vi "Saccade suppression - continuous flash LED by time.vi"() -> ()   [LabVIEW 2013]
uses:
  <vilib>/Platform/TimedLoop/XDataNode/timing_clust.ctl
  <vilib>/Platform/TimedLoop/XDataNode/nitl_modes.ctl
  <vilib>/Platform/TimedLoop/XDataNode/wakeup.ctl
  <vilib>/gmath/statdist.llb/Uniform (Discrete) Random.vi
  Eye tracking dependencies/Global 1.vi
  <vilib>/platform/TimedLoop/XDataNode/XDataNode.xnode
  <vilib>/Platform/TimedLoop/XDataNode/XDNodeRunTimeDep.lvlib
  <vilib>/gmath/NI_Gmath.lvlib
panel:
  out "Eye tracker":bool
  out "Std name":string="70915_animal15-21_exp1"
  out "Blank":bool
  out "Total number of trials":i32=1
  out "Running!":bool
  in  "Location":string="F:\\Beh_Data\\"
  out "File name exists!":bool
  out "Current trial #":u16=1
  out "LED":bool
  in  "Abort":bool caption="run-stop"
  in  "File name":string="18-137_flash"
  in  "Save data":bool
  out "State Missed":bool
  out "VS missed":bool
  out "State busy":bool
  out "VS busy":bool
  in  "Tab Control":T1(tab)=enum."VS Parameters"
  in  "Notes":string
  in  "Start recording @":string
  in  "Inserted probe @":string
  in  "Brain region":string
  in  "Anesthesia @":string
  in  "Anesthesia":string
  in  "Probe configuration":string
  in  "Probe use number":string
  in  "Probe ID":string
  in  "Probe type":string
  in  "Electrode spacing":string
  in  "Electrode area":string
  in  "Penetration angle (to pia)":string
  in  "Penetration coordinates":string
  in  "Penetration distance":string
  in  "Penetration number":string
  in  "Genotype":string
  in  "Transfection":string
  in  "Mass":string
  in  "Sex":string
  in  "Age":string
  in  "Animal ID":string="14-4"
  in  "inter flash interval (ms)":dbl=6000.0
  in  "Max jitter (ms)":dbl=500.0
  in  "VS type":string="saccade_grating"
  in  "Background luminance":sgl=60.0
  in  "Pulse amp 0":sgl
  in  "Pulse amp 1":sgl
  in  "Pulse delay (ms)":sgl
  in  "Pulse width (ms)":sgl
  in  "Pulse period":sgl
  in  "Pulse #":sgl
  in  "LED mode":u16(ring) items=["No LED", "Random"]
  in  "Chance (%)":dbl
  in  "# of trials":i32=1
  in  "run-stop":bool
  in  "Time (min)":sgl=5.0
  in  "Flash luminance":sgl=100.0
  in  "flash duration (ms)":dbl=16.0
  in  "VS subtype":string="shiftByTime2"
  in  "Include blanks":bool
  in  "# of blank trials":i32=6
  in  "INTERLEAVE BLANKS":bool
  in  "Give reward":bool
  in  "Manually give shock":bool
  in  "Water duration (ms)":u32=30
  in  "Shock duration (ms)":u32=10
  in  "Water refractory period (ms)":u32=500
  in  "Shock refractory period (ms)":u32=1000
  in  "Trial timeout (ms)":u32=3000
  in  "Track eye":bool=TRUE
  in  "Allow shock":bool
  in  "Allow timeout":bool
  in  "Manually give water":bool
  in  "Reward period (ms)":u32
  in  "Reward start delay (ms)":u32
  in  "Lick threshold (V)":fxp<+,32,16>=1.600006103515625
  in  "VS threshold (V)":fxp<+,32,16>=2.0
  out "Originating IP":string="192.168.137.2"
  out "Incoming data":string="TrlDone 1.000 "
  in  "Update cycle (ms)":dbl=50.0
  in  "Local IP_This computer":string="192.168.137.10"
  in  "Remote IP_Broadcast":string="192.168.137.255"
  in  "Remote IP_State machine":string="192.168.137.2"
  in  "Remote IP_Visual stimulation":string="192.168.137.3"
  in  "Local port":u16=9090
  in  "Remote port":u16=9091
  out "Error 2":string
  # "Saccade suppression project"
  # "Current trial"
  # "of"
  # "System Status"
  # "VS"
  # "State machine"
  # "Busy"
  # "Missed trial"
  # "Max 20 characters"
  # "(w/o LED)"
  # "Alt: saccade_grating"
  # "Alt: continuous_flash"
  # "movingByTime"
  # "stripeFlipByTime"
  # "gratingFlipByTime"
  # "Time per trial (min)"
  # "MAX 199.9988"
  # "(% of blank trials that have LED)"
  # "Alt: saccade_grating"
  # "shiftByTime"
  # "Errors for debugging"
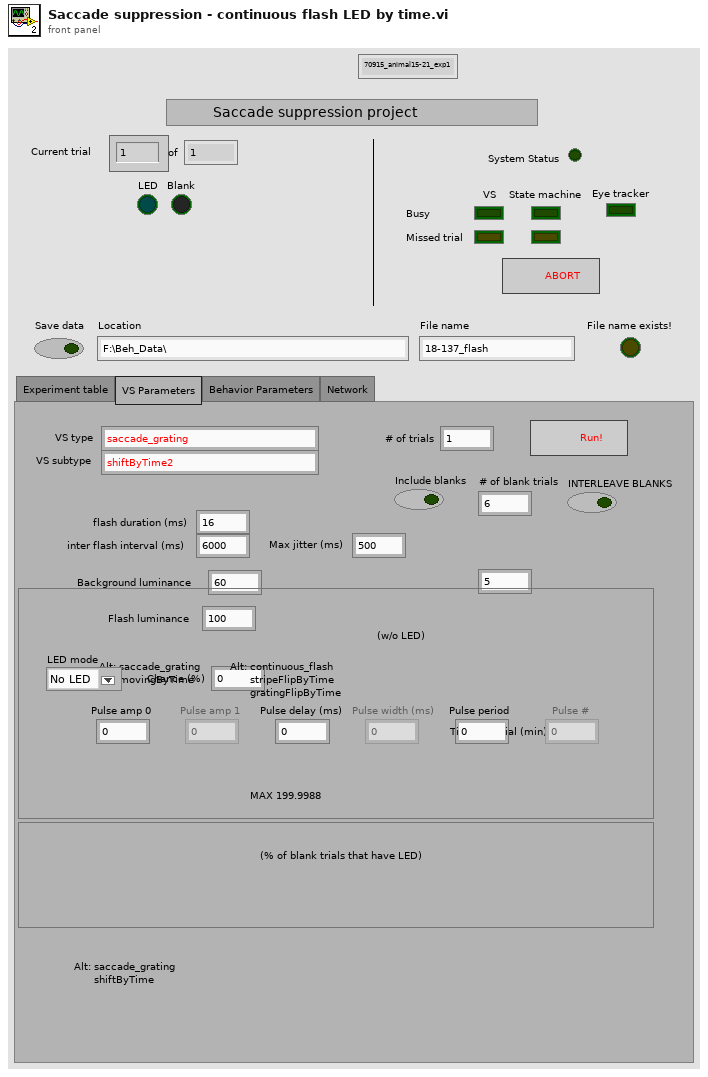
[diagram p1: front panel]
types:
  T1 = enum32{"Experiment table", "VS Parameters", "Behavior Parameters", "Network"}
  T2 = typedef "XDNodeRunTimeDep.lvlib/timing_clust.ctl" = cluster{"Expected End [f-1]":u64, "Actual End [f-1]":u64, "Finished Late? [f-1]":bool, "Expected End [i-1]":u64, "Actual End [i-1]":u64, "Finished Late? [i-1]":bool, "Expected Start [i]":u64, "Actual Start [i]":u64, "Expected Start [f]":u64, "Actual Start [f]":u64, "Source Name":string, "Structure Name":string, "Period":i64, "Deadline":i64, "Offset":i64, "Start":i64, "Priority":i32, "Timeout":i32, "Mode":T3, "Wakeup Reason":T4, "Error":errorcluster, "Source Type":string, "Secondary Source Type":string, "Global End Time":u64, "Global Start Time":u64, "Frame Duration":u64, "Iteration Duration":u64, "Assigned CPU":i32, "I/O Scan Engine Mode":u32}
  T3 = typedef "XDNodeRunTimeDep.lvlib/nitl_modes.ctl" = enum32{"No Change", "Process missed periods, maintain original phase", "Discard missed periods, maintain original phase", "Process missed periods, ignore original phase", "Discard missed periods, ignore original phase"}
  T4 = typedef "XDNodeRunTimeDep.lvlib/wakeup.ctl" = enum32{"Normal", "Aborted", "Asynchronous wakeup", "Timing source error", "Timed loop error", "Timeout"}
  T5 = enum16{"big-endian, network order", "native, host order", "little-endian"}
  T6 = enum16{"open", "replace", "create", "open or create", "replace or create", "replace or create with confirmation"}
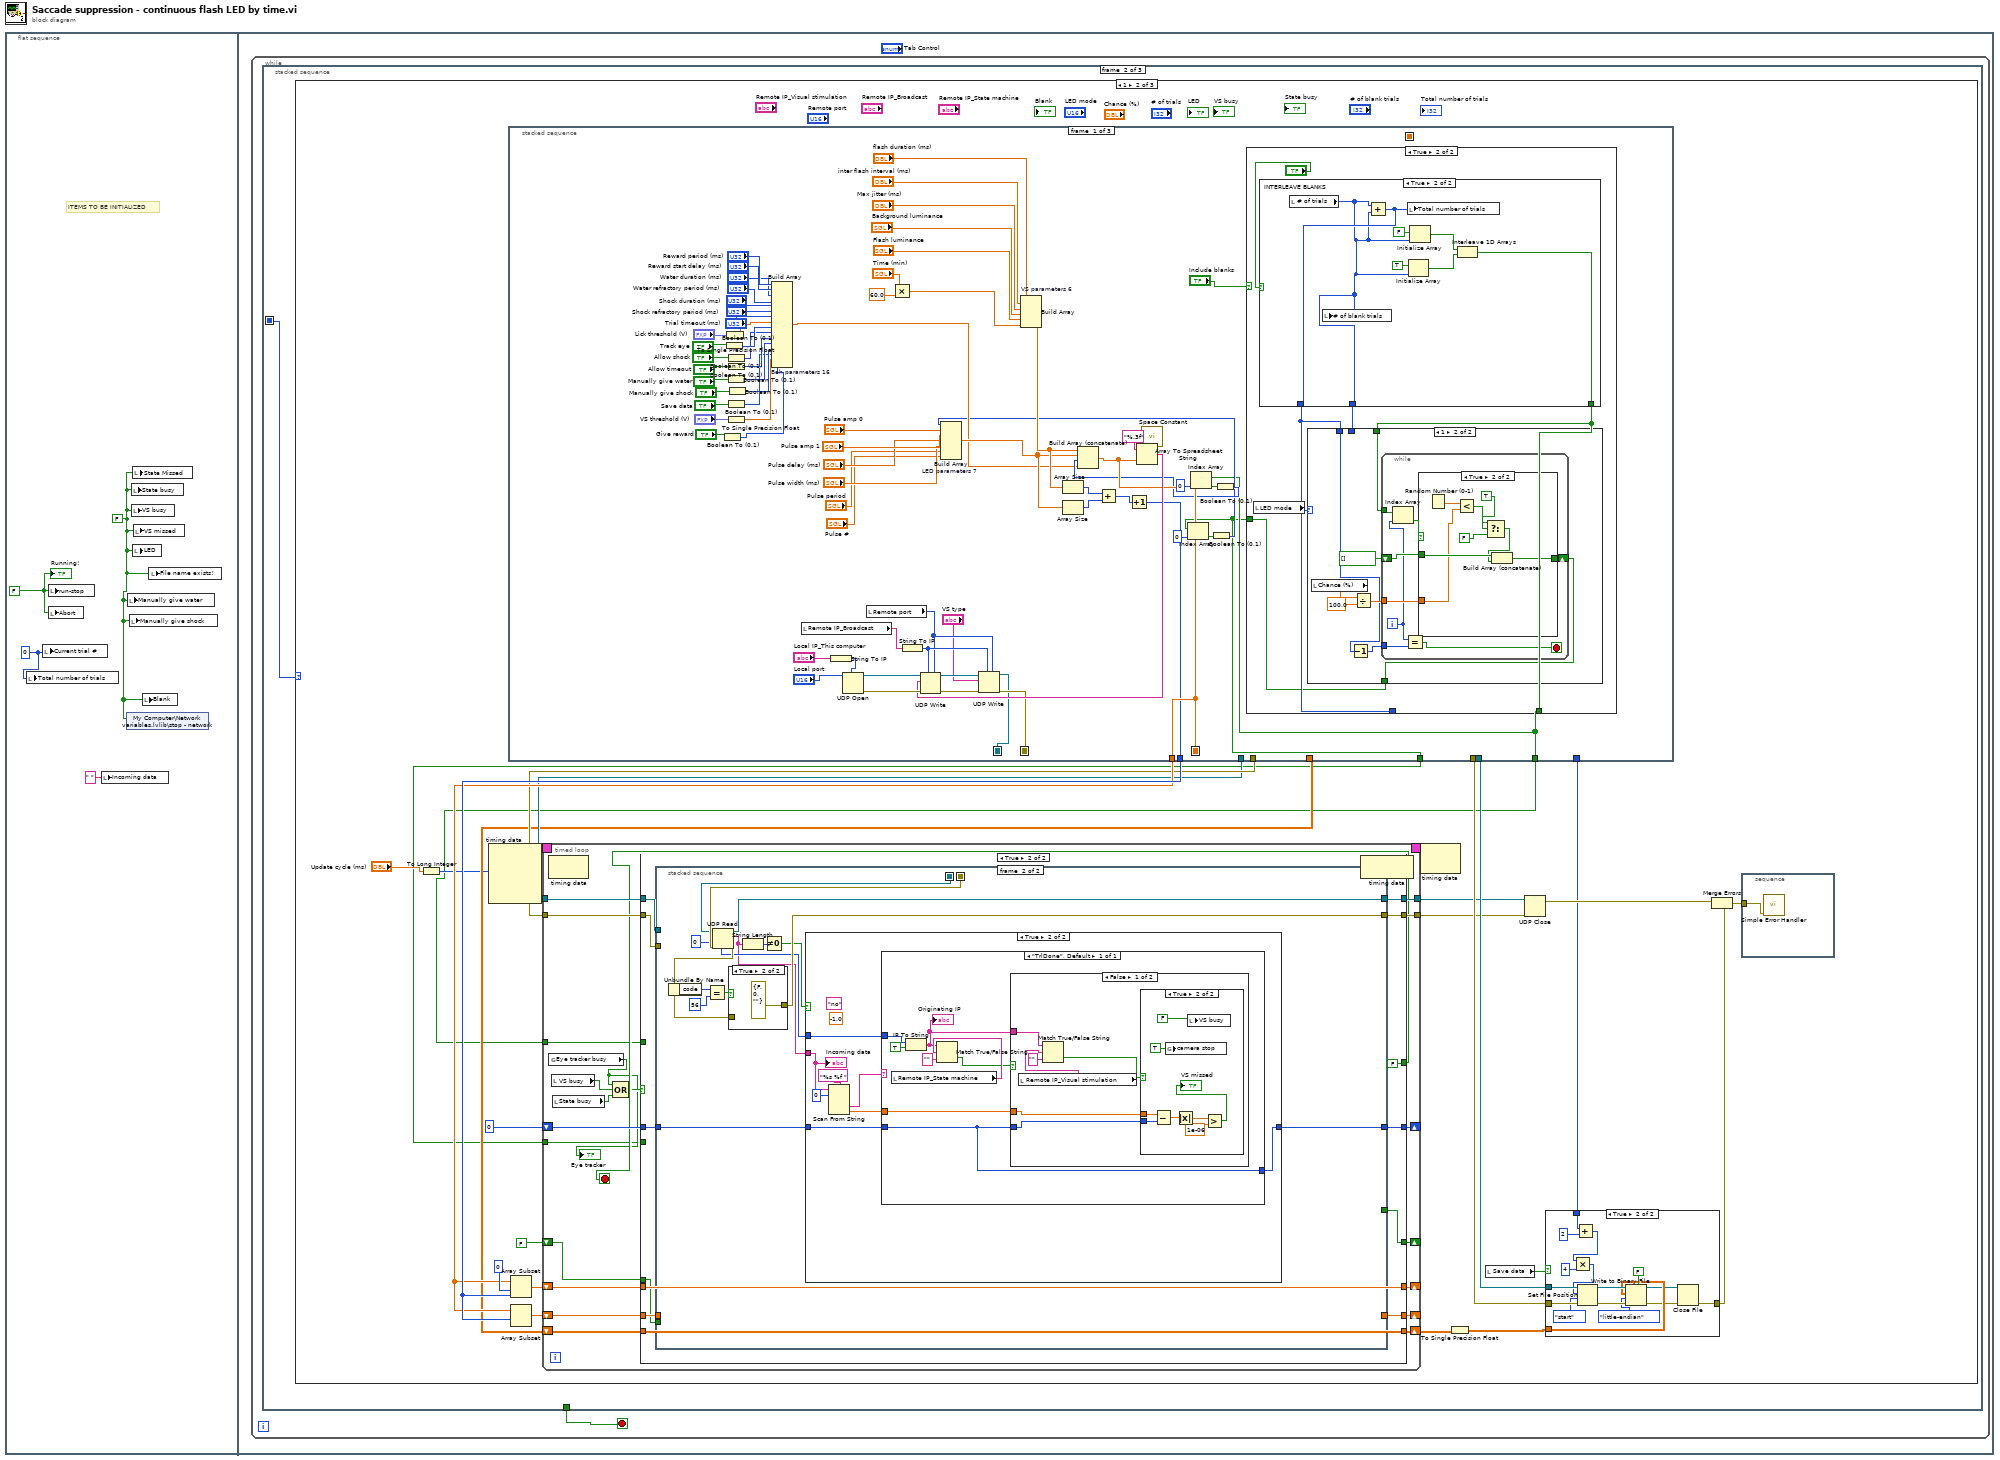
[diagram p0: block diagram]
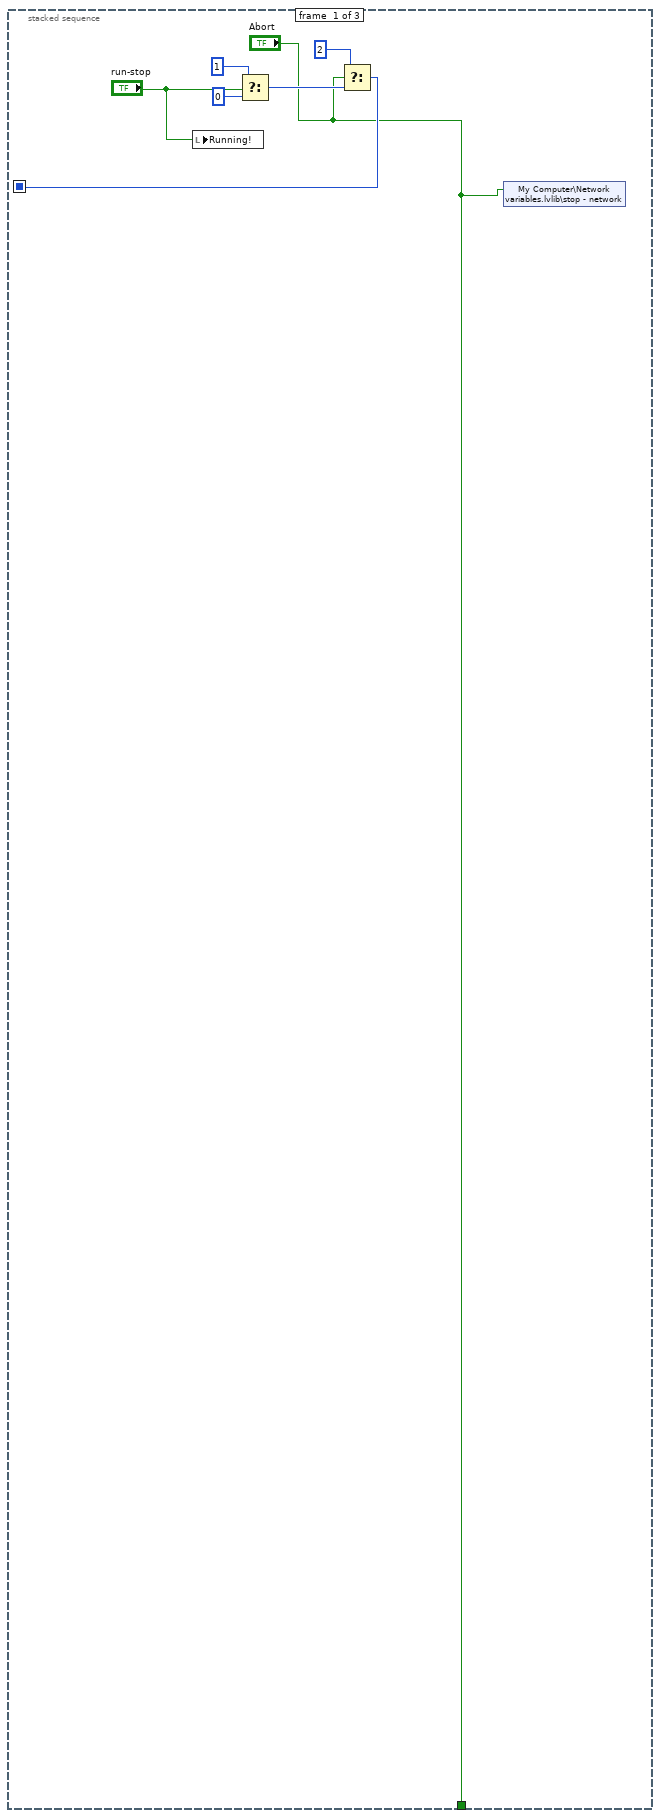
[diagram p2: hidden frame]
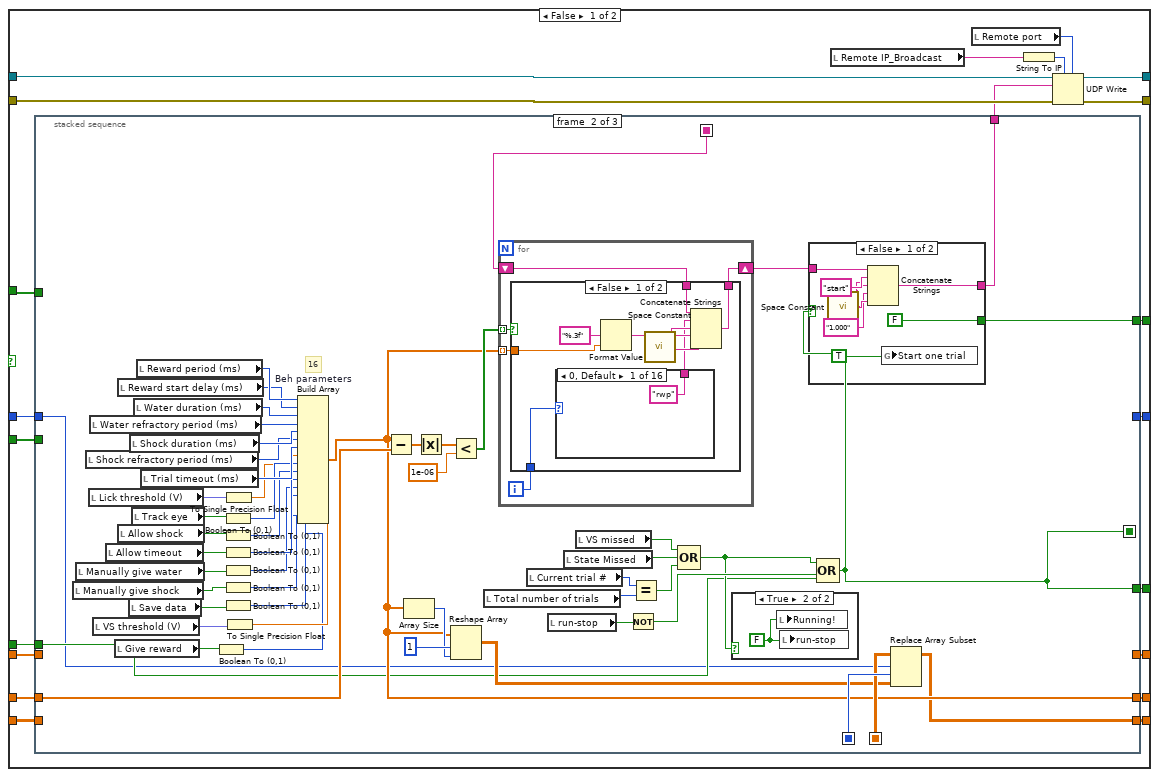
[diagram p4: hidden frame]
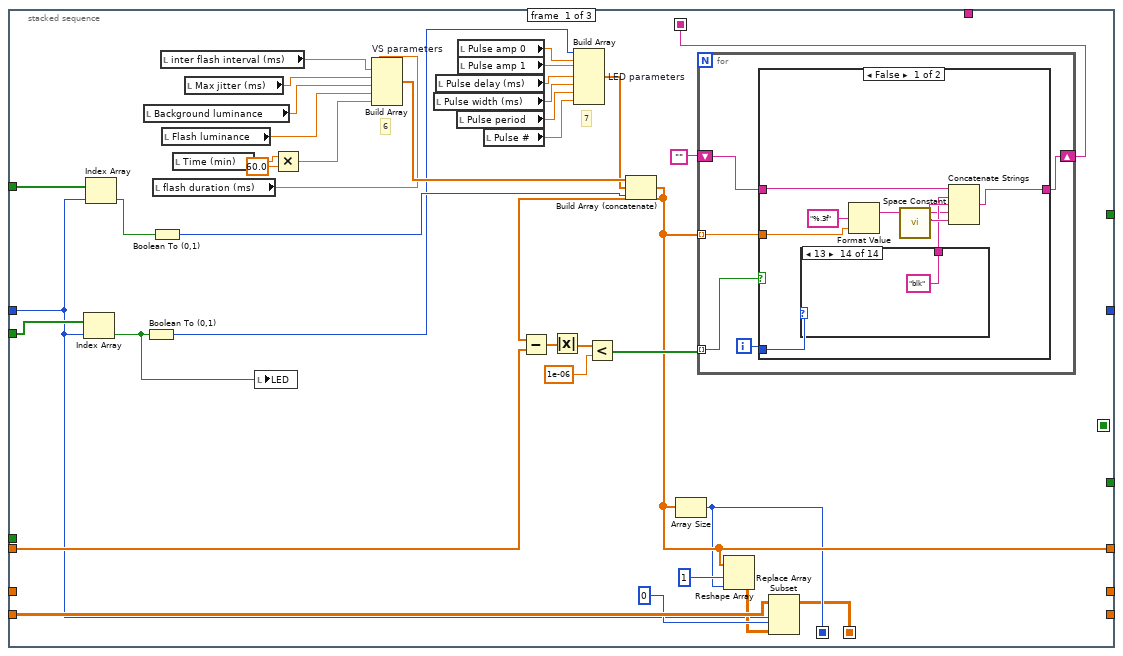
[diagram p5: hidden frame]
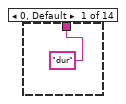
[diagram p6: hidden frame]
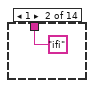
[diagram p7: hidden frame]
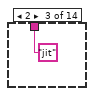
[diagram p8: hidden frame]
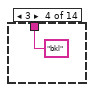
[diagram p9: hidden frame]
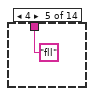
[diagram p10: hidden frame]
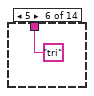
[diagram p11: hidden frame]
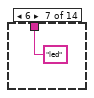
[diagram p12: hidden frame]
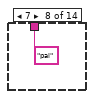
[diagram p13: hidden frame]
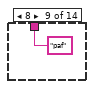
[diagram p14: hidden frame]
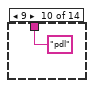
[diagram p15: hidden frame]
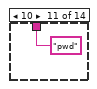
[diagram p16: hidden frame]
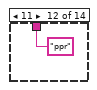
[diagram p17: hidden frame]
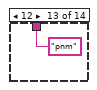
[diagram p18: hidden frame]
diagram:
  n1 = flat-sequence {
    frame #0 {
      w3 = u16 0
      w2 = FALSE ("L dist ind")
      w4 = FALSE
      # "ITEMS TO BE INITIALIZED"
      n2 = local write "Total number of trials"(w3) -> ()
      n3 = local write "Current trial #"(w3) -> ()
      n4 = local write "run-stop"(w4) -> ()
      n5 = local write "Abort"(w4) -> ()
      n6 = local write "Incoming data"(" " ("Incoming data")) -> ()
      n7 = shared-variable "My Computer\\Network variables.lvlib\\stop - network"(w2) -> ()  [unwired: 1 in, 1 out]
      n8 = local write "Manually give water"(w2) -> ()
      n9 = local write "Manually give shock"(w2) -> ()
      n10 = local write "State busy"(w2) -> ()
      n11 = local write "VS busy"(w2) -> ()
      n12 = local write "State Missed"(w2) -> ()
      n13 = local write "LED"(w2) -> ()
      n14 = local write "VS missed"(w2) -> ()
      n15 = local write "Blank"(w2) -> ()
      n16 = local write "File name exists!"(w2) -> ()
      "Running!" <- w4
    }
    frame #1 {
      n17 = while {
        stop <- w5 stop-if-true
        n18 = stacked-sequence {
          seq-local: [w8 _ _] -> [_ w13 _]
          tunnel: ["Abort" _ _] -> w5
          frame #0 {
            n19 = local write "Running!"("run-stop") -> ()
            n20 = Select(t=u8 1, s="run-stop", f=u8 0) -> (s? t:f=w9:u8)
            n21 = Select(t=u8 2, s="Abort", f=w9) -> (s? t:f=w8:u8)
            n22 = shared-variable "My Computer\\Network variables.lvlib\\stop - network"("Abort") -> ()  [unwired: 1 in, 1 out]
          }
          frame #1 {
            n23 = case shown="1" w13 {
              frame 0, Default {
              }
              frame 1 {
                n24 = To Long Integer(number="Update cycle (ms)") -> (32bit integer=w23:i32)
                n25 = node-c288(w23) -> (w40:T2)  [unwired: 3 in]
                n26 = stacked-sequence {
                  seq-local: [w445 _ _] -> [_ _ w627]
                  seq-local: [_ w569 _] -> [_ _ w618]
                  seq-local: [w455 _ _] -> [_ _ w616]
                  seq-local: [w454 _ _] -> [_ _ w602]
                  tunnel: [w445 _ _] -> w35
                  tunnel: [w441 _ _] -> w36
                  tunnel: [_ _ w600] -> w32
                  tunnel: [_ _ w599] -> w31
                  tunnel: [_ _ w621] -> w30
                  tunnel: [_ _ w620] -> w26
                  tunnel: [_ _ w619] -> w25
                  tunnel: [_ _ w597] -> w16
                  tunnel: [w437 _ _] -> w15
                  tunnel: [w436 _ _] -> w14
                  frame #0 {
                    n27 = Boolean To (0,1)(Boolean="Give reward") -> (0, 1=w456:i16)
                    n28 = Boolean To (0,1)(Boolean="Track eye") -> (0, 1=w496:i16)
                    n29 = To Single Precision Float(number="Lick threshold (V)") -> (single precision float=w461:sgl)
                    n30 = Boolean To (0,1)(Boolean="Allow shock") -> (0, 1=w494:i16)
                    n31 = Boolean To (0,1)(Boolean="Allow timeout") -> (0, 1=w492:i16)
                    n32 = Boolean To (0,1)(Boolean="Manually give water") -> (0, 1=w490:i16)
                    n33 = Boolean To (0,1)(Boolean="Save data") -> (0, 1=w487:i16)
                    n34 = To Single Precision Float(number="VS threshold (V)") -> (single precision float=w458:sgl)
                    n35 = Boolean To (0,1)(Boolean="Manually give shock") -> (0, 1=w489:i16)
                    n36 = Build Array "Beh parameters 16"("Reward period (ms)", "Reward start delay (ms)", "Water duration (ms)", "Water refractory period (ms)", "Shock duration (ms)", "Shock refractory period (ms)", "Trial timeout (ms)", w461, w496, w494, w492, w490, w489, w487, w458, w456) -> (w443:sgl[])
                    n37 = local read "Remote IP_Broadcast"() -> (w474:string)
                    n38 = String To IP(1:"Local IP_This computer") -> (0:w478:u32)
                    n39 = UDP Open(7:w478, 11:"Local port") -> (port=w475:refnum<k16>, 0:w479:errorcluster)  [unwired: 3 in, 1 out]
                    n40 = local read "Remote port"() -> (w469:u16)
                    n41 = Multiply(x="Time (min)", y=sgl 60.0) -> (x*y=w434:sgl)
                    n42 = String To IP(1:w474) -> (0:w470:u32)
                    n43 = Build Array "VS parameters 6"("flash duration (ms)", "inter flash interval (ms)", "Max jitter (ms)", "Background luminance", "Flash luminance", w434) -> (w465:dbl[])
                    n44 = Array Size(array=w465) -> (size(s)=w463:i32)
                    n45 = call <vilib>:"Space Constant.vi"() -> ("String"=w472:string)
                    n46 = case shown="True" "Include blanks" {
                      tunnel: [w508 w512] -> w437
                      tunnel: [w506 w514] -> _
                      tunnel: [w505 w513] -> w436
                      frame False {
                        n47 = local read "# of trials"() -> (w506:i32)
                        n48 = Initialize Array(FALSE, w506) -> (w505:bool[])
                        n49 = Initialize Array(FALSE, w506) -> (w508:bool[])
                        n50 = local write "Total number of trials"(w506) -> ()
                      }
                      frame True {
                        n51 = local read "LED mode"() -> (w515:u16)
                        n52 = case shown="True" "INTERLEAVE BLANKS" {
                          tunnel: [w518 w536] -> w514
                          tunnel: [w517 w531] -> w512
                          tunnel: [w516 w534] -> w511
                          frame False {
                            n53 = local read "# of blank trials"() -> (w516:i32)
                            n54 = local read "# of trials"() -> (w519:i32)
                            n55 = Add(x=w519, y=w516) -> (x+y=w518:i32)
                            n56 = local write "Total number of trials"(w518) -> ()
                            n57 = Initialize Array(FALSE, w519) -> (w520:bool[])
                            n58 = for {
                              N: w516 -> [_]
                              shift-right: [w524] -> w517
                              shift-left: w520 -> [w525]
                              n59 = Array Size(array=w525) -> (size(s)=w529:i32)
                              n60 = call-poly <vilib>:"Discrete Random.vi"("n"=w529, "samples"=1) -> ("uniform (discrete) random data"=w528:i32[])  [unwired: 8 in, 1 out]
                              n61 = Index Array(array=w528, index=0) -> (element=w526:i32)
                              n62 = Decrement(x=w526) -> (x-1=w523:i32)
                              n63 = Insert Into Array(array=w525, index=w523, new element=TRUE) -> (w524:bool[])
                            }
                          }
                          frame True {
                            n64 = local read "# of trials"() -> (w534:i32)
                            n65 = local write "# of blank trials"(w534) -> ()
                            n66 = Add(x=w534, y=w534) -> (x+y=w536:i32)
                            n67 = local write "Total number of trials"(w536) -> ()
                            n68 = Initialize Array(TRUE, w534) -> (w532:bool[])
                            n69 = Initialize Array(FALSE, w534) -> (w533:bool[])
                            n70 = Interleave 1D Arrays(w533, w532) -> (w531:bool[])
                          }
                        }
                        n71 = case shown="1" w515 {
                          tunnel: w514 -> [w540 w542]
                          tunnel: [w539 w543] -> w513
                          tunnel: w512 -> [_ w548]
                          tunnel: w511 -> [_ _]
                          frame 0, Default {
                            n72 = Initialize Array(FALSE, w540) -> (w539:bool[])
                          }
                          frame 1 {
                            n73 = local read "Chance (%)"() -> (w546:dbl)
                            n74 = Decrement(x=w542) -> (x-1=w541:i32)
                            n75 = Divide(x=w546, y=100.0) -> (x/y=w544:dbl)
                            n76 = while {
                              tunnel: w548 -> [w556]
                              shift-right: [w554] -> w543
                              shift-left: bool[] [] -> [w553]
                              tunnel: w544 -> [w552]
                              tunnel: w541 -> [w550]
                              i -> [w551]
                              stop <- w549 stop-if-true
                              n77 = Index Array(array=w556, index=w551) -> (element=w555:bool)
                              n78 = Equal?(x=w551, y=w550) -> (x = y?=w549:bool)
                              n79 = case shown="True" w555 {
                                tunnel: [w558 w567] -> w554
                                tunnel: w553 -> [w557 w566]
                                tunnel: w552 -> [_ w561]
                                frame False {
                                n80 = Build Array (concatenate)(w557, FALSE) -> (w558:bool[])
                                }
                                frame True {
                                n81 = Random Number (0-1)() -> (number: 0 to 1=w560:dbl)
                                n82 = Less?(x=w560, y=w561) -> (x < y?=w562:bool)
                                n83 = Select(t=TRUE, s=w562, f=FALSE) -> (s? t:f=w565:bool)
                                n84 = Build Array (concatenate)(w566, w565) -> (w567:bool[])
                                }
                              }
                            }
                          }
                        }
                      }
                    }
                    n85 = Index Array(array=w436, index=0) -> (element=w439:bool)
                    n86 = Index Array(array=w437, index=0) -> (element=w446:bool)
                    n87 = Boolean To (0,1)(Boolean=w439) -> (0, 1=w438:i16)
                    n88 = Build Array "LED parameters 7"(w438, "Pulse amp 0", "Pulse amp 1", "Pulse delay (ms)", "Pulse width (ms)", "Pulse period", "Pulse #") -> (w464:sgl[])
                    n89 = Array Size(array=w464) -> (size(s)=w462:i32)
                    n90 = Add(x=w463, y=w462) -> (x+y=w442:i32)
                    n91 = Increment(x=w442) -> (x+1=w441:i32)
                    n92 = Boolean To (0,1)(Boolean=w446) -> (0, 1=w444:i16)
                    n93 = Build Array (concatenate)(w465, w464, w444, w443) -> (w445:dbl[])
                    n94 = Array To Spreadsheet String(delimiter (Tab)=w472, array=w445, 3:"%.3f" ("format string")) -> (spreadsheet string=w471:string)
                    n95 = UDP Write(address=w470, port or service name=w469, connection ID=w475, data in=w471, 8:w479) -> (error out=w468:errorcluster, 3:w467:refnum<k16>)  [unwired: 1 in]
                    n96 = UDP Write(address=w470, port or service name=w469, connection ID=w467, data in="VS type", 8:w468) -> (error out=w455:errorcluster, 3:w454:refnum<k16>)  [unwired: 1 in]
                  }
                  frame #1 {
                    w576 = "&" ("string")
                    # "state definition"
                    n97 = local read "inter flash interval (ms)"() -> (w591:dbl)
                    n98 = local read "Total number of trials"() -> (w568:i32)
                    n99 = local read "Max jitter (ms)"() -> (w590:dbl)
                    n100 = local read "VS subtype"() -> (w595:string)
                    n101 = local read "Chance (%)"() -> (w589:dbl)
                    n102 = local read "LED mode"() -> (w592:u16)
                    n103 = local read "VS type"() -> (w596:string)
                    n104 = String To Byte Array(string=w596) -> (unsigned byte array=w594:u8[])
                    n105 = String To Byte Array(string=w595) -> (unsigned byte array=w593:u8[])
                    n106 = Concatenate Strings("idle", w576, "vs before", w576, "vs", w576, "vs after", w576, "cycle end", w576, "reward", w576, "reward refractory", w576, "punish", w576, "punish refractory", w576, "exit", w576, "timeout", w576) -> (w577:string)
                    n107 = Build Array (concatenate)(w594, w593, w592, w568, w591, w590, w589) -> (w573:dbl[])
                    n108 = String To Byte Array(string=w577) -> (unsigned byte array=w571:u8[])
                    n109 = Initialize Array(sgl 0.0 ("element"), 37 ("dimension size")) -> (w572:sgl[])
                    n110 = Build Array (concatenate)(w573, w572, w571) -> (w570:dbl[])
                    n111 = To Single Precision Float(number=w570) -> (single precision float=w569:sgl[])
                  }
                  frame #2 {
                    # "# of parameters, column"
                    n112 = local read "Save data"() -> (w624:bool)
                    n113 = local read "Remote IP_Broadcast"() -> (w610:string)
                    n114 = local read "Remote port"() -> (w608:u16)
                    n115 = String To IP(1:w610) -> (0:w609:u32)
                    n116 = local read "Total number of trials"() -> (w617:i32)
                    n117 = Array Size(array=w627) -> (size(s)=w625:i32)
                    n118 = Build Array(w617, w625) -> (w623:i32[])
                    n119 = Initialize Array(sgl 0.0, w617, w625) -> (w621:sgl[][])
                    n120 = To Single Precision Float(number=w623) -> (single precision float=w622:sgl[])
                    n121 = case shown="True" w624 {
                      tunnel: w622 -> [_ w700]
                      tunnel: w621 -> [_ w699]
                      tunnel: [_ w698] -> w620
                      tunnel: [_ w697] -> w619
                      tunnel: w618 -> [_ w696]
                      tunnel: ["" w632] -> w604
                      tunnel: [_ w631] -> w597
                      frame False {
                      }
                      frame True {
                        w667 = 20 ("dimension size")
                        w637 = 500 ("dimension size")
                        w639 = T5."little-endian" ("byte order (0:big-endian, network order)")
                        w709 = enum16{"start", "end", "current"}."start" ("from (0:start)")
                        # "param array"
                        # "row and col\nfor param array"
                        # "first 500 singles for common params"
                        # "reserve 500 singles"
                        # "write behhavior params"
                        # "datapath"
                        n122 = while {
                          tunnel: [w740] -> w702
                          tunnel: [w739] -> w701
                          tunnel: [w732] -> w632
                          stop <- w737 continue-if-true
                          (unwired) "0" ("replace string (\"\")")
                          w761 = "/"
                          n123 = Get Date/Time String() -> (date string=w763:string)  [unwired: 3 in, 1 out]
                          n124 = Match Pattern(string=w763, regular expression=w761) -> (before substring=w760:string, after substring=w762:string)  [unwired: 1 in, 2 out]
                          n125 = Decimal String To Number(string=w760) -> (number=w755:i32)  [unwired: 2 in, 1 out]
                          n126 = Match Pattern(string=w762, regular expression=w761) -> (before substring=w759:string, after substring=w749:string)  [unwired: 1 in, 2 out]
                          n127 = Number To Decimal String(number=w755, width (-)=i16 2) -> (decimal integer string=w757:string)
                          n128 = call <vilib>:"Space Constant.vi"() -> ("String"=w756:string)
                          n129 = Decimal String To Number(string=w759) -> (number=w752:i32)  [unwired: 2 in, 1 out]
                          n130 = Search and Replace String(input string=w757, search string=w756) -> (result string=w747:string)  [unwired: 6 in, 3 out]
                          n131 = Number To Decimal String(number=w752, width (-)=i16 2) -> (decimal integer string=w754:string)
                          n132 = String Subset(string=w749, offset (0)=2) -> (substring=w745:string)  [unwired: 1 in]
                          n133 = call <vilib>:"Space Constant.vi"() -> ("String"=w753:string)
                          n134 = Search and Replace String(input string=w754, search string=w753, replace string="0" ("replace string (\"\")")) -> (result string=w746:string)  [unwired: 5 in, 3 out]
                          n135 = Concatenate Strings(w747, w746, w745) -> (w735:string)
                          n136 = Concatenate Strings(w735, "_" ("string"), "File name") -> (w732:string)
                          "Std name" <- w732
                          n137 = Concatenate Strings("Location", w735, "_" ("string"), "File name", ".be2" ("string")) -> (w742:string)
                          n138 = Wait (ms)(milliseconds to wait=u32 100) -> ()  [unwired: 1 out]
                          n139 = String To Path(string=w742) -> (path=w741:path)
                          n140 = call <vilib>:"Check if File or Folder Exists.vi"("path"=w741) -> ("error out"=w739:errorcluster, "file or folder exists?"=w737:bool, "dup path"=w740:path)  [unwired: 8 in]
                          "File name exists!" <- w737
                        }
                        n141 = String To Byte Array(string="Animal ID") -> (unsigned byte array=w659:u8[])
                        n142 = String To Byte Array(string="Genotype") -> (unsigned byte array=w650:u8[])
                        n143 = String To Byte Array(string="Age") -> (unsigned byte array=w651:u8[])
                        n144 = String To Byte Array(string="Sex") -> (unsigned byte array=w652:u8[])
                        n145 = String To Byte Array(string="Mass") -> (unsigned byte array=w653:u8[])
                        n146 = String To Byte Array(string="Transfection") -> (unsigned byte array=w654:u8[])
                        n147 = String To Byte Array(string="Penetration number") -> (unsigned byte array=w656:u8[])
                        n148 = String To Byte Array(string="Penetration distance") -> (unsigned byte array=w658:u8[])
                        n149 = String To Byte Array(string="Penetration coordinates") -> (unsigned byte array=w682:u8[])
                        n150 = String To Byte Array(string="Penetration angle (to pia)") -> (unsigned byte array=w683:u8[])
                        n151 = String To Byte Array(string="Electrode area") -> (unsigned byte array=w684:u8[])
                        n152 = String To Byte Array(string="Electrode spacing") -> (unsigned byte array=w685:u8[])
                        n153 = String To Byte Array(string="Probe type") -> (unsigned byte array=w686:u8[])
                        n154 = String To Byte Array(string="Probe ID") -> (unsigned byte array=w687:u8[])
                        n155 = String To Byte Array(string="Probe use number") -> (unsigned byte array=w688:u8[])
                        n156 = String To Byte Array(string="Probe configuration") -> (unsigned byte array=w689:u8[])
                        n157 = String To Byte Array(string="Anesthesia") -> (unsigned byte array=w690:u8[])
                        n158 = String To Byte Array(string="Anesthesia @") -> (unsigned byte array=w691:u8[])
                        n159 = String To Byte Array(string="Brain region") -> (unsigned byte array=w692:u8[])
                        n160 = String To Byte Array(string="Inserted probe @") -> (unsigned byte array=w693:u8[])
                        n161 = String To Byte Array(string="Start recording @") -> (unsigned byte array=w694:u8[])
                        n162 = String To Byte Array(string="Notes") -> (unsigned byte array=w695:u8[])
                        n163 = Build Array(w659, w650, w651, w652, w653, w654, w656, w658, w682, w683, w684, w685, w686, w687, w688, w689, w690, w691, w692, w693, w694, w695) -> (w662:u8[][])
                        n164 = for {
                          tunnel: w662 -> [w729] mode=indexing
                          tunnel: [w728] -> w660 mode=indexing
                          tunnel: w667 -> [w727]
                          n165 = Initialize Array(u8 0 ("element"), w727) -> (w731:u8[])
                          n166 = Replace Array Subset(array=w731, new element=w729) -> (w728:u8[])  [unwired: 1 in]
                        }
                        n167 = Array Size(array=w662) -> (size(s)=w664:i32[])
                        n168 = Index Array(array=w664, index=0) -> (element=w666:i32)
                        n169 = Open/Create/Replace File(file path (use dialog)=w702, error in=w701, operation (0:open)=T6."create", access (0:read/write)=enum16{"read/write", "read-only", "write-only"}."write-only") -> (refnum out=w723:refnum<file>, error out=w722:errorcluster)  [unwired: 2 in, 1 out]
                        n170 = Multiply(x=w667, y=w666) -> (x*y=w635:i32)
                        n171 = Set File Position(offset (in bytes) (0)=i64 0, refnum=w723, from (0:start)=w709, error in=w722) -> (refnum out=w643:refnum<file>, error out=w641:errorcluster)
                        n172 = To Single Precision Float(number=w660) -> (single precision float=w661:sgl[][])
                        n173 = Initialize Array(sgl 0.0 ("element"), w637) -> (w719:sgl[])
                        n174 = Reshape Array(w661, 1 ("dimension size"), w635) -> (w638:sgl[][])
                        n175 = Write to Binary File(file (use dialog)=w643, data=w638, error in=w641, 5:FALSE ("prepend array or string size? (T)"), 9:w639) -> (refnum out=w642:refnum<file>, error out=w640:errorcluster)  [unwired: 1 in, 1 out]
                        n176 = Write to Binary File(file (use dialog)=w642, data=w719, error in=w640, 5:FALSE ("prepend array or string size? (T)"), 9:w639) -> (refnum out=w717:refnum<file>, error out=w716:errorcluster)  [unwired: 1 in, 1 out]
                        n177 = Multiply(x=w635, y=4) -> (x*y=w636:i32)
                        n178 = Set File Position(offset (in bytes) (0)=w636, refnum=w717, from (0:start)=w709, error in=w716) -> (refnum out=w715:refnum<file>, error out=w714:errorcluster)
                        n179 = Add(x=w635, y=w637) -> (x+y=w631:i32)
                        n180 = Write to Binary File(file (use dialog)=w715, data=w696, error in=w714, 5:FALSE ("prepend array or string size? (T)"), 9:w639) -> (refnum out=w713:refnum<file>, error out=w712:errorcluster)  [unwired: 1 in, 1 out]
                        n181 = Multiply(x=w631, y=4) -> (x*y=w711:i32)
                        n182 = Set File Position(offset (in bytes) (0)=w711, refnum=w713, from (0:start)=w709, error in=w712) -> (refnum out=w707:refnum<file>, error out=w706:errorcluster)
                        n183 = Write to Binary File(file (use dialog)=w707, data=w700, error in=w706, 5:FALSE ("prepend array or string size? (T)"), 9:w639) -> (refnum out=w705:refnum<file>, error out=w704:errorcluster)  [unwired: 1 in, 1 out]
                        n184 = Write to Binary File(file (use dialog)=w705, data=w699, error in=w704, 5:FALSE ("prepend array or string size? (T)"), 9:w639) -> (refnum out=w697:refnum<file>, error out=w698:errorcluster)  [unwired: 1 in, 1 out]
                      }
                    }
                    n185 = String Length(string=w604) -> (length=w607:i32)
                    n186 = Not Equal To 0?(x=w607) -> (x != 0?=w606:bool)
                    n187 = Select(t=w604, s=w606, f="Test") -> (s? t:f=w603:string)
                    n188 = UDP Write(address=w609, port or service name=w608, connection ID=w602, data in=w603, 8:w616) -> (error out=w615:errorcluster, 3:w601:refnum<k16>)  [unwired: 1 in]
                    n189 = UDP Write(address=w609, port or service name=w608, connection ID=w601, data in="VS subtype", 8:w615) -> (error out=w611:errorcluster, 3:w599:refnum<k16>)  [unwired: 1 in]
                    n190 = Unbundle By Name(w611) -> ("code"=w614:i32)
                    n191 = Equal?(x=w614, y=56) -> (x = y?=w612:bool)
                    n192 = case shown="True" w612 {
                      tunnel: w611 -> [w628 _]
                      tunnel: [w628 errorcluster {"status"=FALSE, "code"=0, "source"=""} ("error out")] -> w600
                      frame False {
                      }
                      frame True {
                      }
                    }
                  }
                }
                n193 = Array Subset(array=w35, index=0, length=w36) -> (w38:dbl[])
                n194 = Array Subset(array=w35, index=w36) -> (w34:dbl[])  [unwired: 1 in]
                n195 = timed-loop {
                  shift-right: [w60] -> _
                  shift-left: u16 0 -> [w59]
                  tunnel: w32 -> [w58]
                  tunnel: w31 -> [w57]
                  tunnel: [w56] -> w17
                  tunnel: [w55] -> w18
                  shift-right: [w54] -> _
                  shift-left: w38 -> [w62]
                  shift-right: [w53] -> _
                  shift-left: w34 -> [w61]
                  shift-right: [w51] -> w29
                  shift-left: w30 -> [w52]
                  shift-right: [w50] -> _
                  shift-left: FALSE -> [w49]
                  timing: w40 -> [_]
                  timing-out: [_] -> w39
                  tunnel: w15 -> [w43]
                  tunnel: w14 -> [w42]
                  stop <- w48 stop-if-true
                  n196 = node-c288() -> ()  [unwired: 1 in, 1 out]
                  n197 = global read "Global 1.vi" "Eye tracker busy"() -> (w44:bool)
                  "Eye tracker" <- w44
                  n198 = local read "VS busy"() -> (w46:bool)
                  n199 = local read "State busy"() -> (w45:bool)
                  n200 = Compound Arithmetic op=OR(w44, w46, w45) -> (w47:bool)
                  n201 = case shown="True" w47 {
                    tunnel: w62 -> [w85 w265]
                    tunnel: w61 -> [w84 w263]
                    tunnel: [w83 w254] -> w60
                    tunnel: w59 -> [w82 w255]
                    tunnel: w58 -> [w78 w261]
                    tunnel: w57 -> [w77 w259]
                    tunnel: [w76 w260] -> w56
                    tunnel: [w75 w258] -> w55
                    tunnel: [w74 w265] -> w54
                    tunnel: [w73 w256] -> w53
                    tunnel: w52 -> [w72 w264]
                    tunnel: [w71 w264] -> w51
                    tunnel: [w70 w257] -> w50
                    tunnel: w49 -> [w69 w262]
                    tunnel: [w67 FALSE] -> w48
                    tunnel: w43 -> [w66 _]
                    tunnel: w42 -> [w65 _]
                    frame False {
                      n202 = stacked-sequence {
                        seq-local: [w109 _ _] -> [_ w176 _]
                        seq-local: [w102 _ _] -> [_ w170 _]
                        seq-local: [w101 _ _] -> [_ w169 _]
                        seq-local: [_ w159 _] -> [_ _ w246]
                        tunnel: w82 -> [w91 w157 w248]
                        tunnel: w85 -> [w114 _ _]
                        tunnel: w84 -> [_ w183 _]
                        tunnel: [_ _ w247] -> w83
                        tunnel: [w106 _ _] -> w74
                        tunnel: [_ w166 _] -> w73
                        tunnel: w72 -> [w105 _ _]
                        tunnel: [_ w164 _] -> w71
                        tunnel: [_ w159 _] -> w70
                        tunnel: w69 -> [_ w160 _]
                        tunnel: [_ w158 _] -> w68
                        tunnel: [_ w151 _] -> w67
                        tunnel: w66 -> [w95 _ _]
                        tunnel: w65 -> [w92 _ _]
                        frame #0 {
                          # "6"
                          # "7"
                          n203 = Index Array(array=w92, index=w91) -> (element=w89:bool)
                          n204 = Index Array(array=w95, index=w91) -> (element=w94:bool)
                          n205 = local read "Background luminance"() -> (w98:sgl)
                          n206 = Boolean To (0,1)(Boolean=w89) -> (0, 1=w90:i16)
                          n207 = Boolean To (0,1)(Boolean=w94) -> (0, 1=w93:i16)
                          n208 = local read "flash duration (ms)"() -> (w96:dbl)
                          n209 = local read "inter flash interval (ms)"() -> (w100:dbl)
                          n210 = local read "Flash luminance"() -> (w97:sgl)
                          n211 = local read "Time (min)"() -> (w87:sgl)
                          n212 = local read "Max jitter (ms)"() -> (w99:dbl)
                          n213 = local write "LED"(w89) -> ()
                          n214 = Multiply(x=w87, y=sgl 60.0) -> (x*y=w88:sgl)
                          n215 = Build Array "VS parameters"(w96, w100, w99, w98, w97, w88) -> (w116:dbl[])
                          n216 = local read "Pulse width (ms)"() -> (w120:sgl)
                          n217 = local read "Pulse delay (ms)"() -> (w119:sgl)
                          n218 = local read "Pulse period"() -> (w121:sgl)
                          n219 = local read "Pulse amp 0"() -> (w117:sgl)
                          n220 = local read "Pulse amp 1"() -> (w118:sgl)
                          n221 = local read "Pulse #"() -> (w122:sgl)
                          n222 = Build Array "LED parameters"(w90, w117, w118, w119, w120, w121, w122) -> (w115:sgl[])
                          n223 = Build Array (concatenate)(w116, w115, w93) -> (w106:dbl[])
                          n224 = Subtract(x=w106, y=w114) -> (x-y=w113:dbl[])
                          n225 = Absolute Value(x=w113) -> (abs(x)=w111:dbl[])
                          n226 = Less?(x=w111, y=1e-06) -> (x < y?=w110:bool[])
                          n227 = Array Size(array=w106) -> (size(s)=w102:i32)
                          n228 = for {
                            tunnel: w110 -> [w127] mode=indexing
                            shift-right: [w125] -> w109
                            shift-left: "" -> [w126]
                            tunnel: w106 -> [w124] mode=indexing
                            i -> [w123]
                            n229 = case shown="False" w127 {
                              tunnel: w126 -> [w135 w150]
                              tunnel: [w134 w150] -> w125
                              tunnel: w123 -> [w132 _]
                              tunnel: w124 -> [w128 _]
                              frame False {
                                n230 = case shown="13" w132 {
                                tunnel: ["dur" "ifi" "jit" "bkl" "fll" "tri" "led" "pai" "paf" "pdl" "pwd" "ppr" "pnm" "blk"] -> w131
                                frame 0, Default {
                                }
                                frame 1 {
                                }
                                frame 2 {
                                }
                                frame 3 {
                                }
                                frame 4 {
                                }
                                frame 5 {
                                }
                                frame 6 {
                                }
                                frame 7 {
                                }
                                frame 8 {
                                }
                                frame 9 {
                                }
                                frame 10 {
                                }
                                frame 11 {
                                }
                                frame 12 {
                                }
                                frame 13 {
                                }
                                }
                                n231 = Format Value(format string="%.3f", value (0)=w128) -> (output string=w129:string)  [unwired: 1 in]
                                n232 = call <vilib>:"Space Constant.vi"() -> ("String"=w133:string)
                                n233 = Concatenate Strings(w135, w131, w133, w129, w133) -> (w134:string)
                              }
                              frame True {
                              }
                            }
                          }
                          n234 = Reshape Array(w106, 1 ("dimension size"), w102) -> (w103:dbl[][])
                          n235 = Replace Array Subset(array=w105, new element=w103, index (row)=w91, index (col)=0) -> (w101:sgl[][])
                        }
                        frame #1 {
                          # "16"
                          n236 = local read "Manually give shock"() -> (w187:bool)
                          n237 = local read "Manually give water"() -> (w189:bool)
                          n238 = local read "Shock refractory period (ms)"() -> (w197:u32)
                          n239 = local read "Lick threshold (V)"() -> (w177:fxp<+,32,16>)
                          n240 = local read "Water refractory period (ms)"() -> (w199:u32)
                          n241 = local read "VS threshold (V)"() -> (w155:fxp<+,32,16>)
                          n242 = local read "Allow timeout"() -> (w191:bool)
                          n243 = local read "Give reward"() -> (w153:bool)
                          n244 = local read "Reward start delay (ms)"() -> (w201:u32)
                          n245 = local read "Allow shock"() -> (w193:bool)
                          n246 = local read "Save data"() -> (w185:bool)
                          n247 = local read "Shock duration (ms)"() -> (w198:u32)
                          n248 = local read "Track eye"() -> (w194:bool)
                          n249 = local read "Water duration (ms)"() -> (w200:u32)
                          n250 = local read "Reward period (ms)"() -> (w202:u32)
                          n251 = local read "Trial timeout (ms)"() -> (w196:u32)
                          n252 = Boolean To (0,1)(Boolean=w153) -> (0, 1=w152:i16)
                          n253 = Boolean To (0,1)(Boolean=w194) -> (0, 1=w195:i16)
                          n254 = Boolean To (0,1)(Boolean=w193) -> (0, 1=w192:i16)
                          n255 = Boolean To (0,1)(Boolean=w191) -> (0, 1=w190:i16)
                          n256 = Boolean To (0,1)(Boolean=w189) -> (0, 1=w188:i16)
                          n257 = Boolean To (0,1)(Boolean=w187) -> (0, 1=w186:i16)
                          n258 = Boolean To (0,1)(Boolean=w185) -> (0, 1=w184:i16)
                          n259 = To Single Precision Float(number=w177) -> (single precision float=w178:sgl)
                          n260 = To Single Precision Float(number=w155) -> (single precision float=w154:sgl)
                          n261 = Build Array "Beh parameters"(w202, w201, w200, w199, w198, w197, w196, w178, w195, w192, w190, w188, w186, w184, w154, w152) -> (w166:sgl[])
                          n262 = Subtract(x=w166, y=w183) -> (x-y=w182:dbl[])
                          n263 = Array Size(array=w166) -> (size(s)=w167:i32)
                          n264 = Absolute Value(x=w182) -> (abs(x)=w180:dbl[])
                          n265 = Less?(x=w180, y=1e-06) -> (x < y?=w179:bool[])
                          n266 = Reshape Array(w166, 1 ("dimension size"), w167) -> (w165:sgl[][])
                          n267 = local read "Total number of trials"() -> (w156:i32)
                          n268 = for {
                            tunnel: w179 -> [w219] mode=indexing
                            tunnel: w166 -> [w218] mode=indexing
                            shift-right: [w216] -> w175
                            shift-left: w176 -> [w217]
                            i -> [w220]
                            n269 = case shown="False" w219 {
                              tunnel: w220 -> [w228 _]
                              tunnel: w218 -> [w226 _]
                              tunnel: w217 -> [w223 w245]
                              tunnel: [w221 w245] -> w216
                              frame False {
                                n270 = case shown="0, Default" w228 {
                                tunnel: ["rwp" "rwd" "wdr" "wre" "shd" "shr" "tto" "lkt" "etk" "ash" "ato" "gwt" "gsh" "sav" "vsh" "rew"] -> w222
                                frame 0, Default {
                                }
                                frame 1 {
                                }
                                frame 2 {
                                }
                                frame 3 {
                                }
                                frame 4 {
                                }
                                frame 5 {
                                }
                                frame 6 {
                                }
                                frame 7 {
                                }
                                frame 8 {
                                }
                                frame 9 {
                                }
                                frame 10 {
                                }
                                frame 11 {
                                }
                                frame 12 {
                                }
                                frame 13 {
                                }
                                frame 14 {
                                }
                                frame 15 {
                                }
                                }
                                n271 = Format Value(format string="%.3f", value (0)=w226) -> (output string=w224:string)  [unwired: 1 in]
                                n272 = call <vilib>:"Space Constant.vi"() -> ("String"=w225:string)
                                n273 = Concatenate Strings(w223, w222, w225, w224, w225) -> (w221:string)
                              }
                              frame True {
                              }
                            }
                          }
                          n274 = local read "Current trial #"() -> (w171:u16)
                          n275 = local read "run-stop"() -> (w163:bool)
                          n276 = local read "State Missed"() -> (w173:bool)
                          n277 = local read "VS missed"() -> (w172:bool)
                          n278 = Not(x=w163) -> (.not. x?=w162:bool)
                          n279 = Equal?(x=w171, y=w156) -> (x = y?=w174:bool)
                          n280 = Compound Arithmetic op=OR(w172, w173, w174) -> (w161:bool)
                          n281 = case shown="True" w161 {
                            frame False {
                            }
                            frame True {
                              w203 = FALSE
                              n282 = local write "Running!"(w203) -> ()
                              n283 = local write "run-stop"(w203) -> ()
                            }
                          }
                          n284 = Compound Arithmetic op=OR(w161, w162, w160) -> (w159:bool)
                          n285 = case shown="False" w159 {
                            tunnel: w175 -> [w210 _]
                            tunnel: [w206 w212] -> w158
                            tunnel: [FALSE TRUE] -> w151
                            frame False {
                              n286 = call <vilib>:"Space Constant.vi"() -> ("String"=w208:string)
                              n287 = Concatenate Strings(w210, "start", w208, "1.000", w208) -> (w206:string)
                              n288 = global write "Global 1.vi" "Start one trial"(TRUE) -> ()
                            }
                            frame True {
                              n289 = call <vilib>:"Space Constant.vi"() -> ("String"=w214:string)
                              n290 = Concatenate Strings("stop", w214, "1.000", w214) -> (w212:string)
                            }
                          }
                          n291 = Replace Array Subset(array=w169, new element=w165, index (row)=w157, index (col)=w170) -> (w164:sgl[][])
                        }
                        frame #2 {
                          n292 = case shown="False" w246 {
                            tunnel: w248 -> [w251 w252]
                            tunnel: [w250 w252] -> w247
                            frame False {
                              w249 = TRUE
                              n293 = Increment(x=w251) -> (x+1=w250:u16)
                              "Current trial #" <- w250
                              n294 = local write "VS busy"(w249) -> ()
                              n295 = local write "State busy"(w249) -> ()
                            }
                            frame True {
                            }
                          }
                        }
                      }
                      n296 = local read "Remote IP_Broadcast"() -> (w79:string)
                      n297 = local read "Remote port"() -> (w81:u16)
                      n298 = String To IP(1:w79) -> (0:w80:u32)
                      n299 = UDP Write(address=w80, port or service name=w81, connection ID=w77, data in=w68, 8:w78) -> (error out=w76:errorcluster, 3:w75:refnum<k16>)  [unwired: 1 in]
                    }
                    frame True {
                      n300 = stacked-sequence {
                        seq-local: [w273 _] -> [_ w369]
                        seq-local: [w272 _] -> [_ w370]
                        tunnel: w263 -> [w289 _]
                        tunnel: w262 -> [w280 _]
                        tunnel: w261 -> [w279 _]
                        tunnel: [_ w364] -> w260
                        tunnel: w259 -> [w278 _]
                        tunnel: [_ w361] -> w258
                        tunnel: [w266 _] -> w257
                        tunnel: [w274 _] -> w256
                        tunnel: w255 -> [_ w358]
                        tunnel: [_ w356] -> w254
                        frame #0 {
                          n301 = local read "Manually give shock"() -> (w299:bool)
                          n302 = local read "Manually give water"() -> (w301:bool)
                          n303 = local read "Shock refractory period (ms)"() -> (w309:u32)
                          n304 = local read "Lick threshold (V)"() -> (w290:fxp<+,32,16>)
                          n305 = local read "Water refractory period (ms)"() -> (w311:u32)
                          n306 = local read "VS threshold (V)"() -> (w270:fxp<+,32,16>)
                          n307 = local read "Allow timeout"() -> (w303:bool)
                          n308 = local read "Reward start delay (ms)"() -> (w313:u32)
                          n309 = local read "Allow shock"() -> (w305:bool)
                          n310 = local read "Save data"() -> (w297:bool)
                          n311 = local read "Shock duration (ms)"() -> (w310:u32)
                          n312 = local read "Track eye"() -> (w306:bool)
                          n313 = local read "Water duration (ms)"() -> (w312:u32)
                          n314 = local read "Reward period (ms)"() -> (w314:u32)
                          n315 = local read "Trial timeout (ms)"() -> (w308:u32)
                          n316 = Boolean To (0,1)(Boolean=w306) -> (0, 1=w307:i16)
                          n317 = Boolean To (0,1)(Boolean=w305) -> (0, 1=w304:i16)
                          n318 = Boolean To (0,1)(Boolean=w303) -> (0, 1=w302:i16)
                          n319 = Boolean To (0,1)(Boolean=w301) -> (0, 1=w300:i16)
                          n320 = Boolean To (0,1)(Boolean=w299) -> (0, 1=w298:i16)
                          n321 = Boolean To (0,1)(Boolean=w297) -> (0, 1=w296:i16)
                          n322 = To Single Precision Float(number=w290) -> (single precision float=w291:sgl)
                          n323 = To Single Precision Float(number=w270) -> (single precision float=w269:sgl)
                          n324 = local read "Give reward"() -> (w268:bool)
                          n325 = Boolean To (0,1)(Boolean=w268) -> (0, 1=w267:i16)
                          n326 = Build Array "Beh parameters"(w314, w313, w312, w311, w310, w309, w308, w291, w307, w304, w302, w300, w298, w296, w269, w267) -> (w274:sgl[])
                          n327 = Subtract(x=w274, y=w289) -> (x-y=w295:dbl[])
                          n328 = Absolute Value(x=w295) -> (abs(x)=w293:dbl[])
                          n329 = Less?(x=w293, y=1e-06) -> (x < y?=w292:bool[])
                          n330 = for {
                            tunnel: w292 -> [w329] mode=indexing
                            tunnel: w274 -> [w328] mode=indexing
                            shift-right: [w326] -> w275
                            shift-left: "" -> [w327]
                            i -> [w330]
                            n331 = case shown="False" w329 {
                              tunnel: w330 -> [w338 _]
                              tunnel: w328 -> [w336 _]
                              tunnel: w327 -> [w333 w355]
                              tunnel: [w331 w355] -> w326
                              frame False {
                                n332 = case shown="15" w338 {
                                tunnel: ["rwp" "rwd" "wdr" "wre" "shd" "shr" "tto" "lkt" "etk" "ash" "ato" "gwt" "gsh" "sav" "vst" "rew"] -> w332
                                frame 0, Default {
                                }
                                frame 1 {
                                }
                                frame 2 {
                                }
                                frame 3 {
                                }
                                frame 4 {
                                }
                                frame 5 {
                                }
                                frame 6 {
                                }
                                frame 7 {
                                }
                                frame 8 {
                                }
                                frame 9 {
                                }
                                frame 10 {
                                }
                                frame 11 {
                                }
                                frame 12 {
                                }
                                frame 13 {
                                }
                                frame 14 {
                                }
                                frame 15 {
                                }
                                }
                                n333 = Format Value(format string="%.3f", value (0)=w336) -> (output string=w334:string)  [unwired: 1 in]
                                n334 = call <vilib>:"Space Constant.vi"() -> ("String"=w335:string)
                                n335 = Concatenate Strings(w333, w332, w335, w334, w335) -> (w331:string)
                              }
                              frame True {
                              }
                            }
                          }
                          n336 = String Length(string=w275) -> (length=w276:i32)
                          n337 = Not Equal To 0?(x=w276) -> (x != 0?=w277:bool)
                          n338 = case shown="True" w277 {
                            tunnel: w279 -> [w315 w321]
                            tunnel: [w315 w320] -> w272
                            tunnel: w278 -> [w316 w319]
                            tunnel: [w316 w318] -> w273
                            tunnel: w275 -> [_ w317]
                            frame False {
                            }
                            frame True {
                              n339 = local read "Remote IP_Broadcast"() -> (w322:string)
                              n340 = local read "Remote port"() -> (w324:u16)
                              n341 = String To IP(1:w322) -> (0:w323:u32)
                              n342 = UDP Write(address=w323, port or service name=w324, connection ID=w319, data in=w317, 8:w321) -> (error out=w320:errorcluster, 3:w318:refnum<k16>)  [unwired: 1 in]
                            }
                          }
                          n343 = local read "Total number of trials"() -> (w271:i32)
                          n344 = local read "Current trial #"() -> (w284:u16)
                          n345 = local read "run-stop"() -> (w283:bool)
                          n346 = local read "State Missed"() -> (w286:bool)
                          n347 = local read "VS missed"() -> (w285:bool)
                          n348 = Not(x=w283) -> (.not. x?=w282:bool)
                          n349 = Equal?(x=w284, y=w271) -> (x = y?=w287:bool)
                          n350 = Compound Arithmetic op=OR(w285, w286, w287) -> (w281:bool)
                          n351 = Compound Arithmetic op=OR(w281, w282, w280) -> (w266:bool)
                          n352 = case shown="True" w266 {
                            frame False {
                            }
                            frame True {
                              w325 = FALSE
                              n353 = local write "Running!"(w325) -> ()
                              n354 = local write "run-stop"(w325) -> ()
                            }
                          }
                        }
                        frame #1 {
                          n355 = UDP Read(connection ID=w369, timeout ms (25000)=0, 8:w370) -> (data out=w357:string, error out=w365:errorcluster, 3:w361:refnum<k16>, 6:w359:u32)  [unwired: 1 in, 1 out]
                          n356 = Unbundle By Name(w365) -> ("code"=w366:i32)
                          n357 = Equal?(x=w366, y=56) -> (x = y?=w368:bool)
                          n358 = case shown="True" w368 {
                            tunnel: w365 -> [w410 _]
                            tunnel: [w410 errorcluster {"status"=FALSE, "code"=0, "source"=""} ("error out")] -> w364
                            frame False {
                            }
                            frame True {
                            }
                          }
                          n359 = String Length(string=w357) -> (length=w363:i32)
                          n360 = Not Equal To 0?(x=w363) -> (x != 0?=w362:bool)
                          n361 = case shown="True" w362 {
                            tunnel: w359 -> [_ w375]
                            tunnel: w358 -> [w371 w374]
                            tunnel: w357 -> [_ w379]
                            tunnel: [w371 w372] -> w356
                            frame False {
                            }
                            frame True {
                              (unwired) -1.0 ("default value 2")
                              (unwired) "no" ("default value 1")
                              n362 = Scan From String(format string="%s %f ", input string=w379, initial scan location=u32 0) -> (output 1=w376:string, output 2=w373:dbl)  [unwired: 3 in, 3 out]
                              n363 = case shown="\"TrlDone\", Default" w376 {
                                tunnel: w375 -> [w387]
                                tunnel: w374 -> [w380]
                                tunnel: w373 -> [w382]
                                tunnel: [w380] -> w372
                                frame "TrlDone", Default {
                                n364 = local read "Remote IP_State machine"() -> (w384:string)
                                n365 = IP To String(1:TRUE ("dot notation? (F)"), 2:w387) -> (0:w381:string)
                                "Originating IP" <- w381
                                n366 = Match True/False String(2:"" ("false string"), 3:w384, 4:w381) -> (0:w383:bool)  [unwired: 1 out]
                                n367 = case shown="False" w383 {
                                tunnel: w380 -> [w388 w407]
                                tunnel: w382 -> [w389 w408]
                                tunnel: w381 -> [w393 _]
                                frame False {
                                n368 = local read "Remote IP_Visual stimulation"() -> (w391:string)
                                n369 = Match True/False String(2:"" ("false string"), 3:w391, 4:w393) -> (0:w390:bool)  [unwired: 1 out]
                                n370 = case shown="True" w390 {
                                tunnel: w389 -> [_ w398]
                                tunnel: w388 -> [_ w397]
                                frame False {
                                "Error 2" <- "Unknown source Error"
                                }
                                frame True {
                                n371 = Subtract(x=w398, y=w397) -> (x-y=w401:dbl)
                                n372 = global write "Global 1.vi" "camera stop"(TRUE ("dot notation? (F)")) -> ()
                                n373 = Absolute Value(x=w401) -> (abs(x)=w400:dbl)
                                n374 = local write "VS busy"(FALSE) -> ()
                                n375 = Greater?(x=w400, y=1e-06) -> (0:→"VS missed":bool)
                                }
                                }
                                }
                                frame True {
                                n376 = Subtract(x=w408, y=w407) -> (x-y=w406:dbl)
                                n377 = local write "State busy"(FALSE) -> ()
                                n378 = Absolute Value(x=w406) -> (abs(x)=w405:dbl)
                                n379 = Greater?(x=w405, y=1e-06) -> (0:→"State Missed":bool)
                                }
                                }
                                }
                              }
                              "Incoming data" <- w379
                            }
                          }
                        }
                      }
                    }
                  }
                  n380 = node-c288() -> ()  [unwired: 1 in, 1 out]
                }
                n381 = node-c288(w39) -> ()  [unwired: 1 out]
                n382 = To Single Precision Float(number=w29) -> (single precision float=w24:sgl[][])
                n383 = local read "Save data"() -> (w27:bool)
                n384 = UDP Close(connection ID=w18, 8:w17) -> (error out=w22:errorcluster)  [unwired: 1 out]
                n385 = case shown="True" w27 {
                  tunnel: w26 -> [w416 w432]
                  tunnel: w25 -> [_ w431]
                  tunnel: w24 -> [_ w423]
                  tunnel: [w416 w420] -> w21
                  tunnel: w16 -> [_ w419]
                  frame False {
                  }
                  frame True {
                    n386 = Add(x=w419, y=2) -> (x+y=w417:i32)
                    n387 = Multiply(x=w417, y=4) -> (x*y=w428:i32)
                    n388 = Set File Position(offset (in bytes) (0)=w428, refnum=w431, from (0:start)=enum16{"start", "end", "current"}."start", error in=w432) -> (refnum out=w425:refnum<file>, error out=w426:errorcluster)
                    n389 = Write to Binary File(file (use dialog)=w425, data=w423, error in=w426, 5:FALSE ("prepend array or string size? (T)"), 9:T5."little-endian" ("byte order (0:big-endian, network order)")) -> (refnum out=w421:refnum<file>, error out=w422:errorcluster)  [unwired: 1 in, 1 out]
                    n390 = Close File(refnum=w421, error in=w422) -> (error out=w420:errorcluster)  [unwired: 1 out]
                  }
                }
                n391 = Merge Errors(w22, w21) -> (w20:errorcluster)
                n392 = stacked-sequence {
                  tunnel: w20 -> [w41]
                  frame #0 {
                    n393 = call <vilib>:"Simple Error Handler.vi"("error in (no error)"=w41) -> ()  [unwired: 4 in, 5 out]
                  }
                }
              }
              frame 2 {
              }
            }
          }
          frame #2 {
            n394 = Wait (ms)(milliseconds to wait=u32 100) -> ()  [unwired: 1 out]
          }
        }
      }
    }
  }
